vi "Cleaning&Misc.vi"() -> ()   [LabVIEW 2014, in "Panels.lvlib"]
uses:
  Panels.lvlib
  CSlibraries-extern/DimLVEvent/DimIndicators/DimIndicators.lvlib
  CS_Core/CSSystem/CoreLib/CoreLib.lvlib
  CSlibraries/UtilityLib/UtilityLib.valueStatus.ctl
  CSlibraries/UtilityLib/UtilityLib.lvlib
  CSlibraries-extern/DimLVEvent/LVDimInterface/LVDimInterface.lvlib
  CS_Core/CSSystem/CoreLib/CoreLib.short 2 byte array.vi
  CS_Core/BaseProcess/BaseProcess.descriptor string definition.ctl
  CS_Core/BaseProcess/BaseProcess.lvlib
  CS_Core/CSSystem/CoreDefs/CoreDefs.rawDataType.ctl
  CS_Core/CSSystem/CoreDefs/CoreDefs.call_type.ctl
  CSlibraries-extern/DimLVEvent/DimIndicators/DimIndicators.numericType.ctl
panel:
  in  "PGSwitch_MonData":T1={"data"=32767.0, "no link"=FALSE, "quality"=1, "timeStamp"=3262371343.476}
  in  "PGSwitch_SetData":T1
  in  "PGSwitch":bool
  in  "call cluster in":T2={"Object"="", "Selector"="", "CallType"=enum."synchronous", "Async Object"="", "Async Selector"="", "Data Descriptor"="", "Data"=[], "Error #"=0, "Expire"=0}
  in  "MRClean6":bool
  in  "MRClean5":bool
  in  "MRClean4":bool
  in  "MRClean3":bool
  in  "MRClean2":bool
  in  "MRClean1":bool
  in  "GCBeamG":bool
  in  "TISBeamG":bool
  in  "BOB6switch":bool
  in  "BOB5switch":bool
  in  "ExcPolarity":bool
  in  "GCBeamG_SetData":T1
  in  "MRClean6_MonData":T1={"data"=32767.0, "no link"=FALSE, "quality"=1, "timeStamp"=3262371343.476}
  out "i ref out":refnum<vi>
  in  "ExcPolarity_SetData":T1
  in  "MRClean5_SetData":T1
  in  "MRClean4_SetData":T1
  in  "MRClean3_SetData":T1
  in  "MRClean2_SetData":T1
  in  "MRClean1_SetData":T1
  in  "TISBeamG_SetData":T1
  in  "BOB6switch_SetData":T1
  in  "BOB5switch_SetData":T1
  in  "MRClean6_SetData":T1
  in  "MRClean5_MonData":T1={"data"=32767.0, "no link"=FALSE, "quality"=1, "timeStamp"=3262371343.476}
  in  "MRClean4_MonData":T1={"data"=32767.0, "no link"=FALSE, "quality"=1, "timeStamp"=3262371343.476}
  in  "MRClean3_MonData":T1={"data"=32767.0, "no link"=FALSE, "quality"=1, "timeStamp"=3262371343.476}
  in  "MRClean2_MonData":T1={"data"=32767.0, "no link"=FALSE, "quality"=1, "timeStamp"=3262371343.476}
  in  "MRClean1_MonData":T1={"data"=32767.0, "no link"=FALSE, "quality"=1, "timeStamp"=3262371343.46}
  in  "GCBeamG_MonData":T1={"data"=32767.0, "no link"=FALSE, "quality"=1, "timeStamp"=3262371343.46}
  in  "TISBeamG_MonData":T1={"data"=3.0, "no link"=FALSE, "quality"=3, "timeStamp"=3262371343.46}
  in  "BOB6switch_MonData":T1={"data"=32767.0, "no link"=FALSE, "quality"=1, "timeStamp"=3262371343.46}
  in  "BOB5switch_MonData":T1={"data"=32767.0, "no link"=FALSE, "quality"=1, "timeStamp"=3262371343.46}
  in  "ExcPolarity_MonData":T1={"data"=3.0, "no link"=FALSE, "quality"=3, "timeStamp"=3262371343.46}
  # "off - cyclotron\non - dipole"
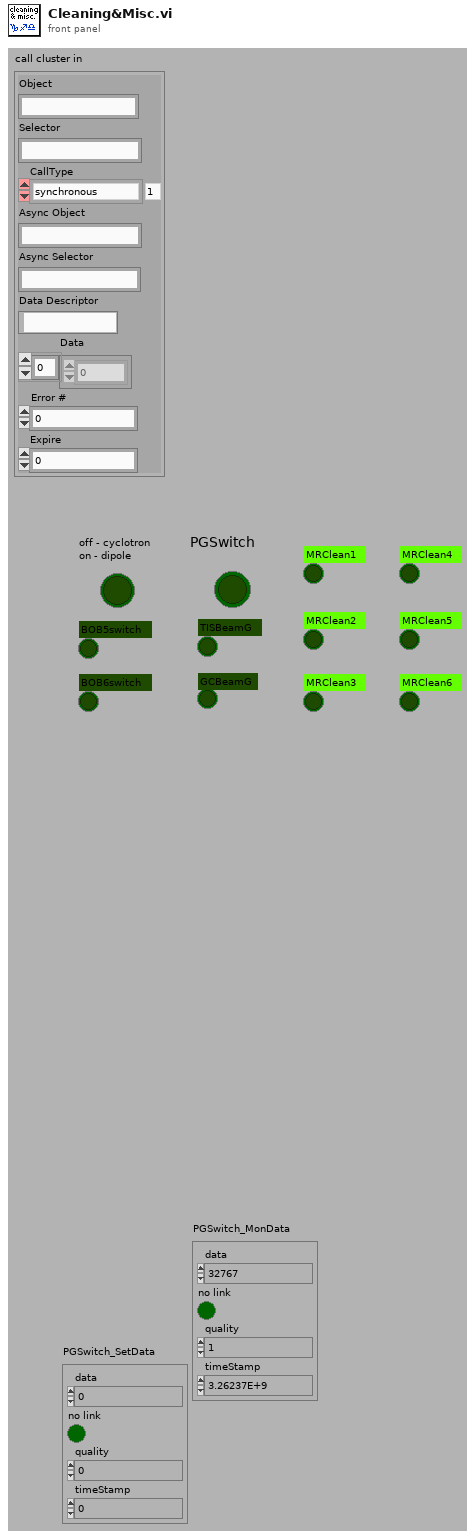
[diagram p1: front panel]
types:
  T1 = typedef "DimIndicators.lvlib/DimIndicators.numericType.ctl" = cluster{"data":dbl, "no link":bool, "quality":i32, "timeStamp":dbl}
  T2 = typedef "CoreDefs.call_type.ctl" = cluster{"Object":string, "Selector":string, "CallType":enum16{"simple", "synchronous", "asynchronous"}, "Async Object":string, "Async Selector":string, "Data Descriptor":T3, "Data":T4, "Error #":i32, "Expire":u32}
  T3 = typedef "BaseProcess.lvlib/BaseProcess.descriptor string definition.ctl" = string
  T4 = typedef "CoreDefs.rawDataType.ctl" = i8[]
  T5 = typedef "UtilityLib.lvlib/UtilityLib.valueStatus.ctl" = enum16{"no info available", "stand by/off", "on", "warning", "alarm/malfunction", "not implemented", "user action required", "important information", "system default", "control default", "indicator default", "button default"}
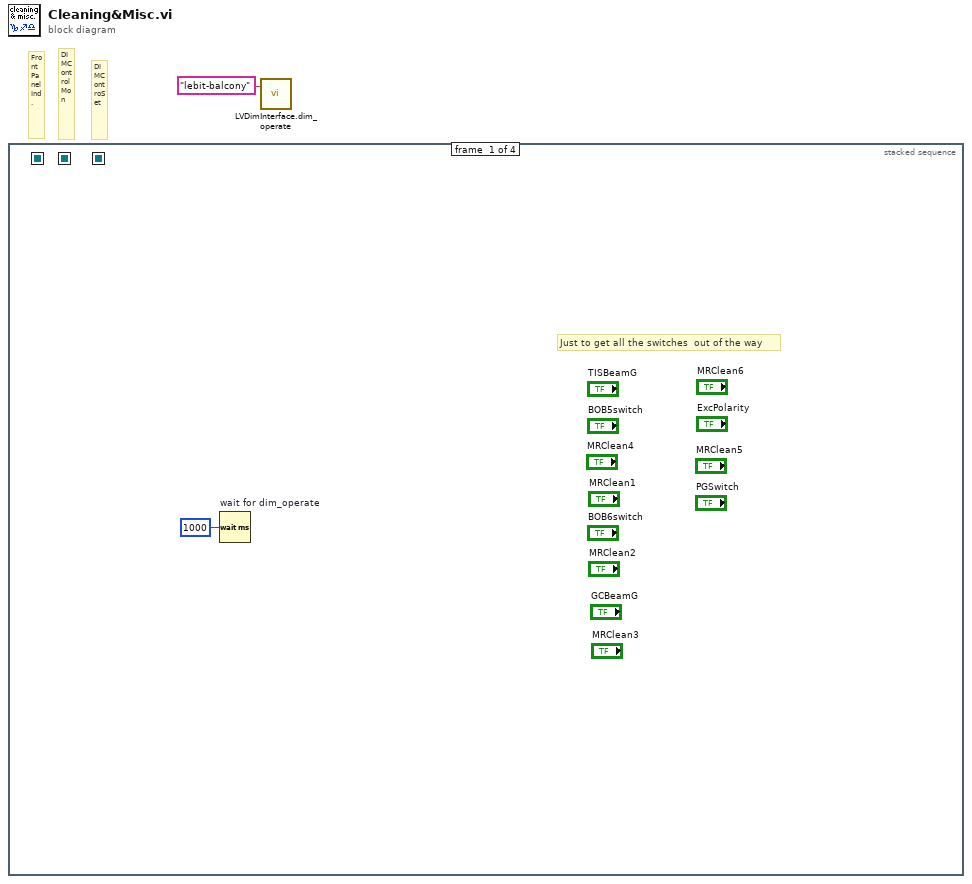
[diagram p0: block diagram]
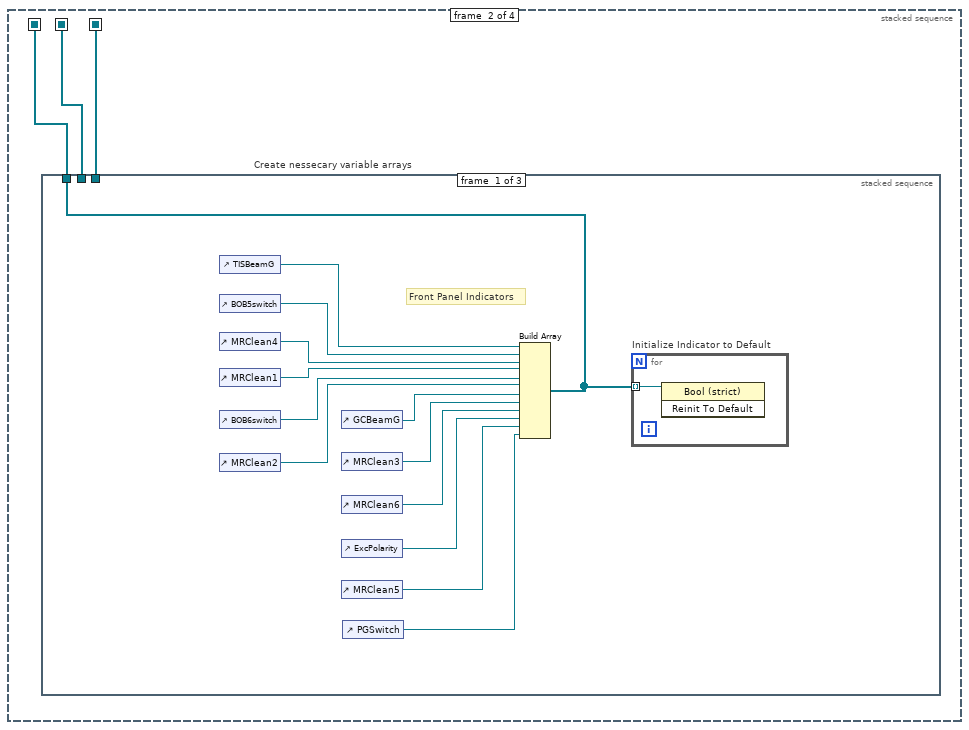
[diagram p2: hidden frame]
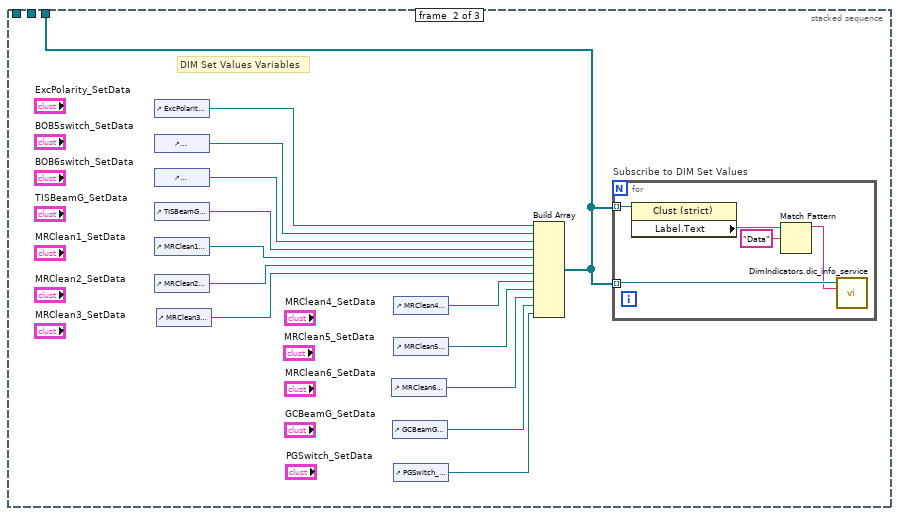
[diagram p3: hidden frame]
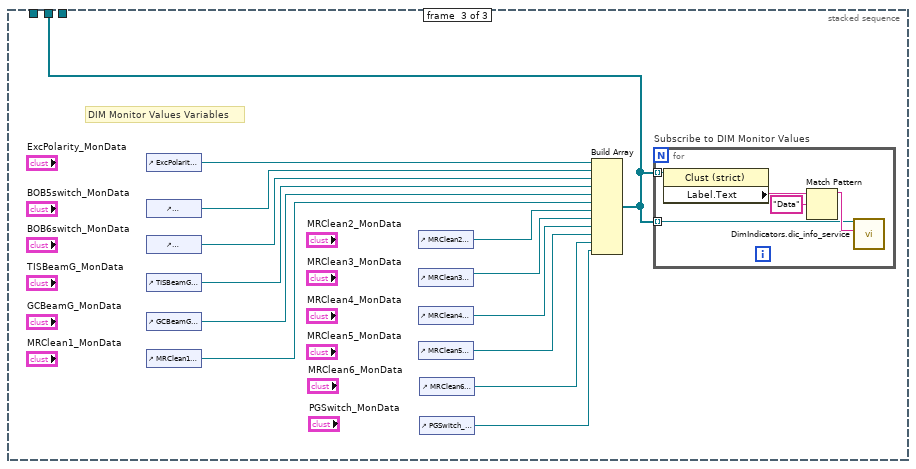
[diagram p4: hidden frame]
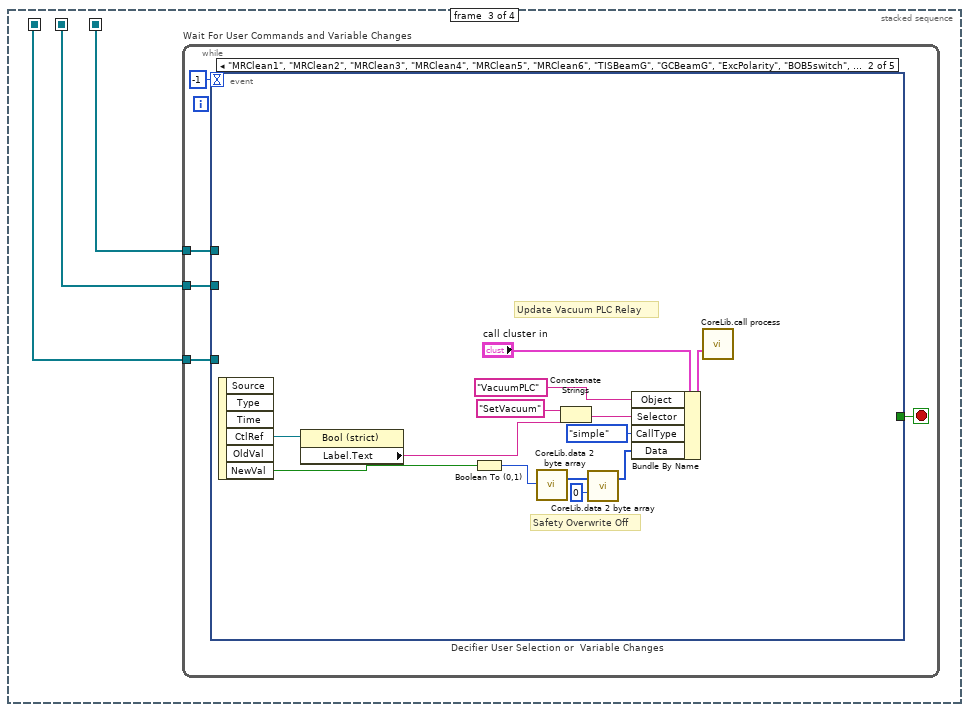
[diagram p5: hidden frame]
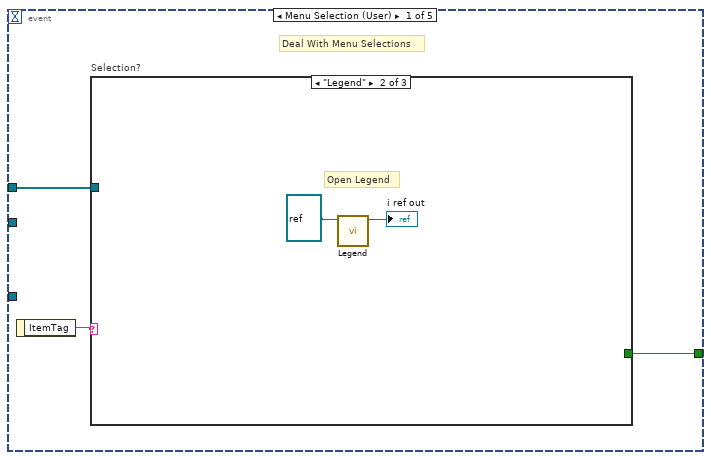
[diagram p6: hidden frame]
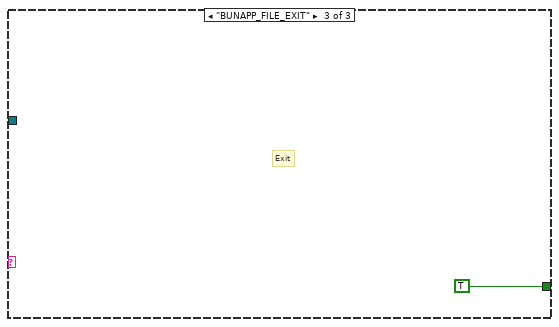
[diagram p8: hidden frame]
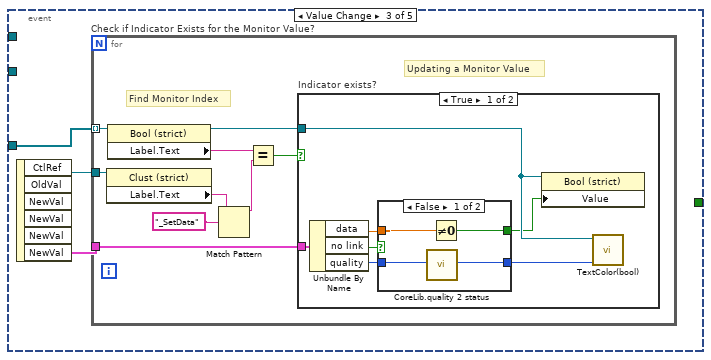
[diagram p9: hidden frame]
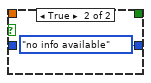
[diagram p10: hidden frame]
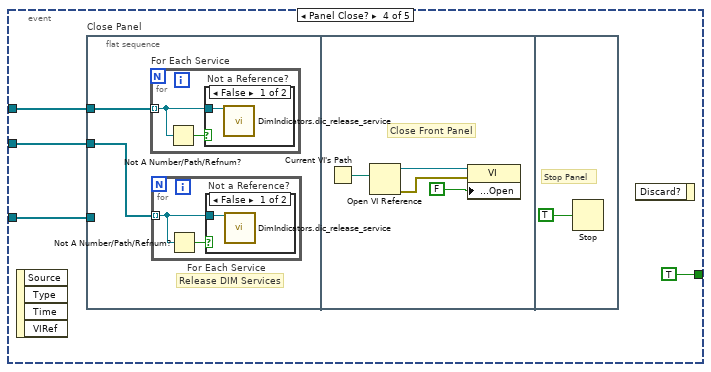
[diagram p12: hidden frame]
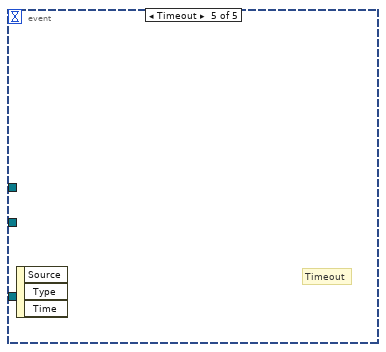
[diagram p15: hidden frame]
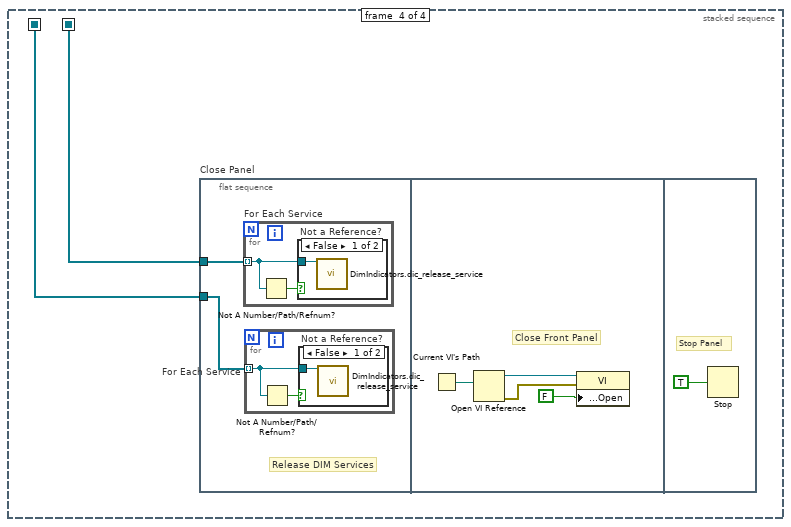
[diagram p16: hidden frame]
diagram:
  # "Front Panel Ind."
  # "DIMControSet"
  # "DIMControlMon"
  n1 = stacked-sequence {
    seq-local: [_ w4 _ _] -> [_ _ w58 w124]
    seq-local: [_ w3 _ _] -> [_ _ w57 w125]
    seq-local: [_ w5 _ _] -> [_ _ w56 _]
    frame #0 {
      # "Just to get all the switches  out of the way"
      n2 = Wait (ms) "wait for dim_operate"(milliseconds to wait=u32 1000) -> ()  [unwired: 1 out]
    }
    frame #1 {
      n3 = stacked-sequence "Create nessecary variable arrays" {
        tunnel: [w7 _ _] -> w5
        tunnel: [_ _ w39] -> w4
        tunnel: [_ w21 _] -> w3
        frame #0 {
          # "Front Panel Indicators"
          n4 = control-ref of="TISBeamG"() -> (w18:refnum<vi>)
          n5 = control-ref of="BOB5switch"() -> (w17:refnum<vi>)
          n6 = control-ref of="MRClean4"() -> (w16:refnum<vi>)
          n7 = control-ref of="MRClean1"() -> (w15:refnum<vi>)
          n8 = control-ref of="BOB6switch"() -> (w14:refnum<vi>)
          n9 = control-ref of="MRClean2"() -> (w13:refnum<vi>)
          n10 = control-ref of="GCBeamG"() -> (w12:refnum<vi>)
          n11 = control-ref of="MRClean3"() -> (w11:refnum<vi>)
          n12 = control-ref of="MRClean6"() -> (w10:refnum<vi>)
          n13 = control-ref of="ExcPolarity"() -> (w9:refnum<vi>)
          n14 = control-ref of="MRClean5"() -> (w8:refnum<vi>)
          n15 = control-ref of="PGSwitch"() -> (w6:refnum<vi>)
          n16 = Build Array(w18, w17, w16, w15, w14, w13, w12, w11, w10, w9, w8, w6) -> (w7:refnum<vi>[])
          n17 = for "Initialize Indicator to Default" {
            tunnel: w7 -> [w19] mode=indexing
            n18 = invoke class="Bool (strict)" method="Reinit To Default"(reference=w19) -> ()  [unwired: 2 in, 3 out]
          }
        }
        frame #1 {
          # "DIM Set Values Variables"
          n19 = control-ref of="ExcPolarity_SetData"() -> (w32:refnum<vi>)
          n20 = control-ref of="BOB5switch_SetData"() -> (w31:refnum<vi>)
          n21 = control-ref of="BOB6switch_SetData"() -> (w30:refnum<vi>)
          n22 = control-ref of="TISBeamG_SetData"() -> (w29:refnum<vi>)
          n23 = control-ref of="MRClean1_SetData"() -> (w28:refnum<vi>)
          n24 = control-ref of="MRClean2_SetData"() -> (w27:refnum<vi>)
          n25 = control-ref of="MRClean3_SetData"() -> (w26:refnum<vi>)
          n26 = control-ref of="MRClean6_SetData"() -> (w23:refnum<vi>)
          n27 = control-ref of="GCBeamG_SetData"() -> (w22:refnum<vi>)
          n28 = control-ref of="MRClean4_SetData"() -> (w25:refnum<vi>)
          n29 = control-ref of="MRClean5_SetData"() -> (w24:refnum<vi>)
          n30 = control-ref of="PGSwitch_SetData"() -> (w20:refnum<vi>)
          n31 = Build Array(w32, w31, w30, w29, w28, w27, w26, w25, w24, w23, w22, w20) -> (w21:refnum<vi>[])
          n32 = for "Subscribe to DIM Set Values" {
            tunnel: w21 -> [w33] mode=indexing
            tunnel: w21 -> [w37] mode=indexing
            n33 = property class="Clust (strict)"(reference=w33) -> ("Label.Text"=w36:string)  [unwired: 1 in, 2 out]
            n34 = Match Pattern(string=w36, regular expression="Data") -> (before substring=w34:string)  [unwired: 1 in, 3 out]
            n35 = call "DimIndicators.dic_info_service.vi"("controlRef"=w37, "serviceName"=w34) -> ()  [unwired: 16 in, 2 out]
          }
        }
        frame #2 {
          # "DIM Monitor Values Variables"
          n36 = control-ref of="ExcPolarity_MonData"() -> (w49:refnum<vi>)
          n37 = control-ref of="BOB5switch_MonData"() -> (w48:refnum<vi>)
          n38 = control-ref of="BOB6switch_MonData"() -> (w47:refnum<vi>)
          n39 = control-ref of="TISBeamG_MonData"() -> (w46:refnum<vi>)
          n40 = control-ref of="GCBeamG_MonData"() -> (w45:refnum<vi>)
          n41 = control-ref of="MRClean1_MonData"() -> (w44:refnum<vi>)
          n42 = control-ref of="MRClean2_MonData"() -> (w43:refnum<vi>)
          n43 = control-ref of="MRClean3_MonData"() -> (w50:refnum<vi>)
          n44 = control-ref of="MRClean4_MonData"() -> (w42:refnum<vi>)
          n45 = control-ref of="MRClean5_MonData"() -> (w41:refnum<vi>)
          n46 = control-ref of="MRClean6_MonData"() -> (w40:refnum<vi>)
          n47 = control-ref of="PGSwitch_MonData"() -> (w38:refnum<vi>)
          n48 = Build Array(w49, w48, w47, w46, w45, w44, w43, w50, w42, w41, w40, w38) -> (w39:refnum<vi>[])
          n49 = for "Subscribe to DIM Monitor Values" {
            tunnel: w39 -> [w52] mode=indexing
            tunnel: w39 -> [w51] mode=indexing
            n50 = property class="Clust (strict)"(reference=w51) -> ("Label.Text"=w54:string)  [unwired: 1 in, 2 out]
            n51 = Match Pattern(string=w54, regular expression="Data") -> (before substring=w53:string)  [unwired: 1 in, 3 out]
            n52 = call "DimIndicators.dic_info_service.vi"("controlRef"=w52, "serviceName"=w53) -> ()  [unwired: 16 in, 2 out]
          }
        }
      }
    }
    frame #2 {
      n53 = while "Wait For User Commands and Variable Changes" {
        tunnel: w58 -> [w62]
        tunnel: w57 -> [w61]
        tunnel: w56 -> [w59]
        stop <- w63 stop-if-true
        n54 = event "Decifier User Selection or  Variable Changes" shown="[1] \"MRClean1\", \"MRClean2\", \"MRClean3\", \"MRClean4\", \"MRClean5\", \"MRClean6\", \"TISBeamG\", \"GCBeamG\", \"ExcPolarity\", \"BOB5switch\", \"BOB6switch\", \"PGSwitch\": Value Change" {
          selector: _ -> [_ _ _ _ _]
          dyn-events: _ -> [_ _ _ _ _]
          timeout: -1 -> [_ _ _ _ _]
          tunnel: [w64 _ _ TRUE ("stop") _] -> w63
          tunnel: w62 -> [_ _ _ w108 _]
          tunnel: w61 -> [w65 _ _ w109 _]
          tunnel: w59 -> [_ _ w84 w107 _]
          event Menu Selection (User) {
            # "Deal With Menu Selections"
            n55 = event-data() -> ("ItemTag"=w66:string)  [unwired: 1 in]
            n56 = case "Selection?" shown="\"Legend\"" w66 {
              tunnel: w65 -> [_ _ _]
              tunnel: [_ _ TRUE ("stop")] -> w64
              frame "False", Default {
              }
              frame "Legend" {
                # "Open Legend"
                n57 = call "Legend.vi"("i ref in"=refnum<vi> refnum) -> ("i ref out"=→"i ref out":refnum<vi>)  [unwired: 10 in]
              }
              frame "BUNAPP_FILE_EXIT" {
                # "Exit"
              }
            }
          }
          event "MRClean1", "MRClean2", "MRClean3", "MRClean4", "MRClean5", "MRClean6", "TISBeamG", "GCBeamG", "ExcPolarity", "BOB5switch", "BOB6switch", "PGSwitch": Value Change {
            # "Safety Overwrite Off"
            # "Update Vacuum PLC Relay"
            n58 = event-data() -> ("CtlRef"=w76:refnum<vi>, "NewVal"=w74:bool)  [unwired: 1 in, 4 out]
            n59 = property class="Bool (strict)"(reference=w76) -> ("Label.Text"=w75:string)  [unwired: 1 in, 2 out]
            n60 = Boolean To (0,1)(Boolean=w74) -> (0, 1=w73:i16)
            n61 = call-poly "CoreLib.data 2 byte array.vi"("i16"=w73) -> ("byteArray out"=w72:T4)  [unwired: 18 in]
            n62 = Concatenate Strings("SetVacuum" ("string"), w75) -> (w78:string)
            n63 = call-poly "CoreLib.data 2 byte array.vi"("byteArray"=w72, "i16"=i16 0) -> ("byteArray out"=w70:T4)  [unwired: 17 in]
            n64 = Bundle By Name(cluster="call cluster in", "Object"="VacuumPLC", "Selector"=w78, "CallType"=enum16{"simple", "synchronous", "asynchronous"}."simple", "Data"=w70) -> (w81:T2)
            n65 = call "CoreLib.call process.vi"("call cluster in"=w81) -> ()  [unwired: 13 in, 2 out]
          }
          event Value Change {
            n66 = event-data() -> ("CtlRef"=w85:refnum<vi>, "NewVal"=w83:T1)  [unwired: 1 in, 4 out]
            n67 = for "Check if Indicator Exists for the Monitor Value?" {
              tunnel: w83 -> [w94]
              tunnel: w84 -> [w91] mode=indexing
              tunnel: w85 -> [w90]
              # "Find Monitor Index"
              # "Updating a Monitor Value"
              n68 = property class="Clust (strict)"(reference=w90) -> ("Label.Text"=w92:string)  [unwired: 1 in, 2 out]
              n69 = property class="Bool (strict)"(reference=w91) -> (reference out=w86:refnum<vi>, "Label.Text"=w88:string)  [unwired: 1 in, 1 out]
              n70 = Match Pattern(string=w92, regular expression="_SetData") -> (before substring=w87:string)  [unwired: 1 in, 3 out]
              n71 = Equal?(x=w88, y=w87) -> (x = y?=w89:bool)
              n72 = case "Indicator exists?" shown="True" w89 {
                tunnel: w94 -> [w101 _]
                tunnel: w86 -> [w96 _]
                frame True {
                  n73 = Unbundle By Name(w101) -> ("data"=w98:dbl, "no link"=w99:bool, "quality"=w100:i32)
                  n74 = case shown="False" w99 {
                    tunnel: w100 -> [w105 _]
                    tunnel: [w104 UtilityLib.valueStatus."no info available" ("valueStatus")] -> w97
                    tunnel: w98 -> [w102 _]
                    tunnel: [w103 _] -> w95
                    frame False {
                      n75 = call "CoreLib.quality 2 status.vi"("quality"=w105) -> ("valueStatus"=w104:T5)  [unwired: 18 in]
                      n76 = Not Equal To 0?(x=w102) -> (x != 0?=w103:bool)
                    }
                    frame True {
                    }
                  }
                  n77 = property on="Property Node" class="Bool (strict)"(reference=w96, "Value"=w95) -> ()  [unwired: 1 in, 2 out]
                  n78 = call "TextColor(bool).vi"("valueStatus"=w97, "Ref"=w96) -> ()  [unwired: 10 in]
                }
                frame False {
                }
              }
            }
          }
          event Panel Close? {
            n79 = event-data() -> ()  [unwired: 1 in, 4 out]
            n80 = flat-sequence "Close Panel" {
              tunnel: w109 -> [w112]
              tunnel: w108 -> [w111]
              tunnel: w107 -> [_]
              frame #0 {
                # "Release DIM Services"
                n81 = for "For Each Service" {
                  tunnel: w112 -> [w117] mode=indexing
                  n82 = Not A Number/Path/Refnum?(number/path/refnum=w117) -> (NaN/Path/Refnum?=w116:bool)
                  n83 = case "Not a Reference?" shown="False" w116 {
                    tunnel: w117 -> [w118 _]
                    frame False {
                      n84 = call "DimIndicators.dic_release_service.vi"("controlRef"=w118) -> ()  [unwired: 18 in, 1 out]
                    }
                    frame True {
                    }
                  }
                }
                n85 = for "For Each Service" {
                  tunnel: w111 -> [w114] mode=indexing
                  n86 = Not A Number/Path/Refnum?(number/path/refnum=w114) -> (NaN/Path/Refnum?=w113:bool)
                  n87 = case "Not a Reference?" shown="False" w113 {
                    tunnel: w114 -> [w115 _]
                    frame False {
                      n88 = call "DimIndicators.dic_release_service.vi"("controlRef"=w115) -> ()  [unwired: 18 in, 1 out]
                    }
                    frame True {
                    }
                  }
                }
              }
              frame #1 {
                # "Close Front Panel"
                n89 = Current VI's Path() -> (path=w120:path)
                n90 = Open VI Reference(vi path=w120) -> (vi reference=w122:refnum<vi>, error out=w119:errorcluster)  [unwired: 5 in]
                n91 = property class="VI"(reference=w122, error in=w119, "Front Panel Window:Open"=FALSE) -> ()  [unwired: 2 out]
              }
              frame #2 {
                # "Stop Panel"
                n92 = Stop(stop? (T)=TRUE) -> ()
              }
            }
            n93 = event-data() -> ()  [unwired: 2 in, 1 out]
          }
          event Timeout {
            # "Timeout"
            n94 = event-data() -> ()  [unwired: 1 in, 3 out]
          }
        }
      }
    }
    frame #3 {
      n95 = flat-sequence "Close Panel" {
        tunnel: w125 -> [w127]
        tunnel: w124 -> [w126]
        frame #0 {
          # "Release DIM Services"
          n96 = for "For Each Service" {
            tunnel: w127 -> [w132] mode=indexing
            n97 = Not A Number/Path/Refnum?(number/path/refnum=w132) -> (NaN/Path/Refnum?=w131:bool)
            n98 = case "Not a Reference?" shown="False" w131 {
              tunnel: w132 -> [w133 _]
              frame False {
                n99 = call "DimIndicators.dic_release_service.vi"("controlRef"=w133) -> ()  [unwired: 18 in, 1 out]
              }
              frame True {
              }
            }
          }
          n100 = for "For Each Service" {
            tunnel: w126 -> [w129] mode=indexing
            n101 = Not A Number/Path/Refnum?(number/path/refnum=w129) -> (NaN/Path/Refnum?=w128:bool)
            n102 = case "Not a Reference?" shown="False" w128 {
              tunnel: w129 -> [w130 _]
              frame False {
                n103 = call "DimIndicators.dic_release_service.vi"("controlRef"=w130) -> ()  [unwired: 18 in, 1 out]
              }
              frame True {
              }
            }
          }
        }
        frame #1 {
          # "Close Front Panel"
          n104 = Current VI's Path() -> (path=w134:path)
          n105 = Open VI Reference(vi path=w134) -> (vi reference=w136:refnum<vi>, error out=w137:errorcluster)  [unwired: 5 in]
          n106 = property class="VI"(reference=w136, error in=w137, "Front Panel Window:Open"=FALSE) -> ()  [unwired: 2 out]
        }
        frame #2 {
          # "Stop Panel"
          n107 = Stop(stop? (T)=TRUE) -> ()
        }
      }
    }
  }
  n108 = call "LVDimInterface.dim_operate.vi"("DNSNode"="lebit-balcony" ("DNS node")) -> ()  [unwired: 19 in]
